vi "Send Return Value.vi"(8 "error in (no error)":errorcluster, 9 "Return Value":variant, 10 "Call in":refnum<class "Call.lvclass">, 11 "Node in":refnum<class "PyObject.lvclass">) -> (0 "error out":errorcluster, 3 "Node out":refnum<class "PyObject.lvclass">)   [LabVIEW 2013, in "JKI_Python_Bridge_for_LV.lvlib" / "PyObject.lvclass"]
uses:
  PyObject.lvclass
  Call/Call.lvclass
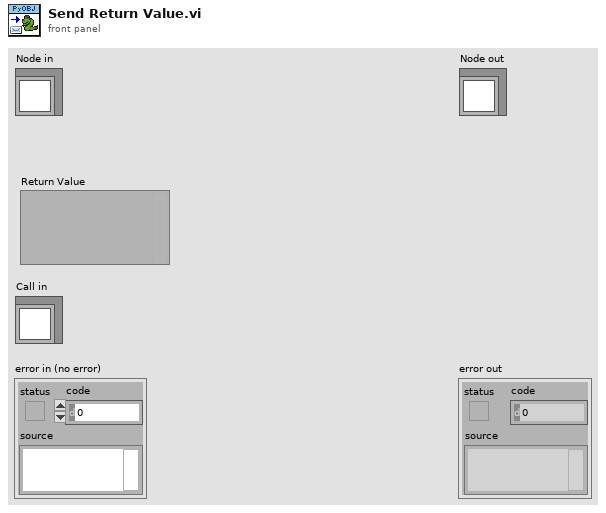
[diagram p1: front panel]
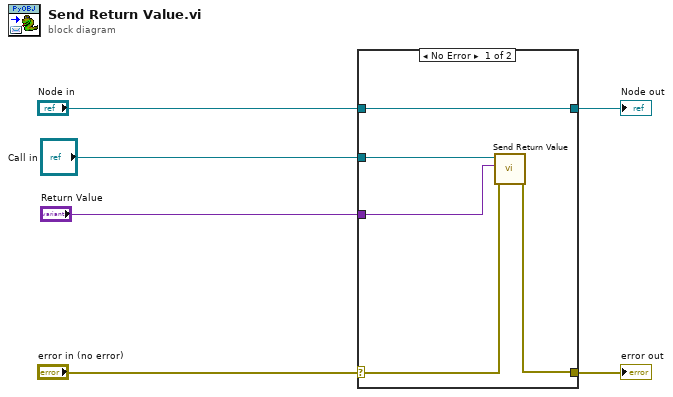
[diagram p0: block diagram]
diagram:
  n1 = case shown="No Error" "error in (no error)" {
    selector: "error in (no error)" -> [w8 w13]
    tunnel: [w7 w13] -> w5
    tunnel: [w11 w12] -> w3
    tunnel: "Node in" -> [w11 w12]
    tunnel: "Return Value" -> [w9 _]
    tunnel: "Call in" -> [w10 _]
    frame No Error {
      n2 = call "Send Return Value.vi"("error in (no error)"=w8, "Return Value"=w9, "Response in"=w10) -> ("error out"=w7:errorcluster)  [unwired: 8 in]
    }
    frame Error {
    }
  }
  "error out" <- w5
  "Node out" <- w3
